vi "Write Saving.vi"(8 "error in (no error)":errorcluster, 10 "Saving":bool, 11 "Saving File Message in":refnum<class "Saving File Message.lvclass">) -> (0 "error out":errorcluster, 3 "Saving File Message out":refnum<class "Saving File Message.lvclass">)   [LabVIEW 2017, in "File Library.lvlib" / "Saving File Message.lvclass"]
uses:
  Saving File Message.lvclass
  Saving File Message.lvclass/Saving File Message.ctl
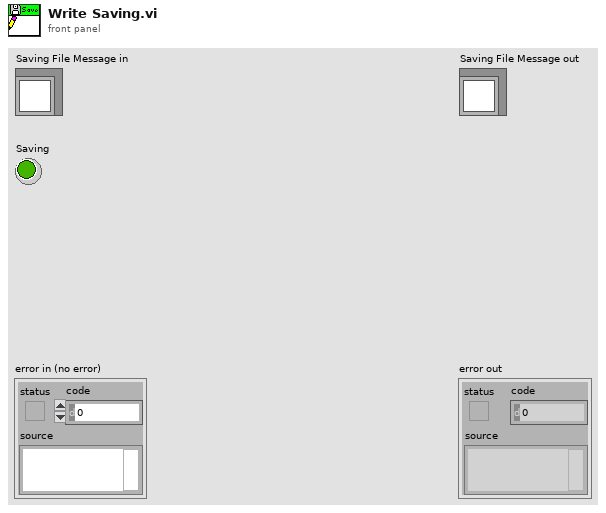
[diagram p1: front panel]
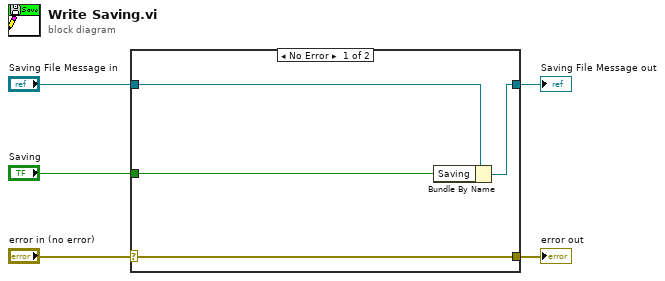
[diagram p0: block diagram]
diagram:
  n1 = case shown="No Error" "error in (no error)" {
    selector: "error in (no error)" -> [w9 w10]
    tunnel: [w9 w10] -> w4
    tunnel: [w7 w11] -> w2
    tunnel: "Saving File Message in" -> [w8 w11]
    tunnel: "Saving" -> [w6 _]
    frame No Error {
      n2 = Bundle By Name(cluster=w8, "Saving"=w6) -> (w7:refnum<class "Saving File Message.lvclass">)
    }
    frame Error {
    }
  }
  "error out" <- w4
  "Saving File Message out" <- w2
